vi "GetLeCroy_SynthFocus_25.vi"(1 "Digitizer Settings":T4={"Digitizer delay (us) "=0.0, "rf points per line"=2048, "lines per plane"=128, "Samp Rate (Hz)"=100000000.0, "Additional dig delay (us)"=0.0, "Voltage Scale"=0.4, "Pre-Looks"=0, "Offset delay (us)"=0.0, "bits A/D"=8, "Avg Num"=1, "DigTimeOut"=5.0, "Rel Dig Delay"=0.0, "Dig Ch"=0, "LeCroyCluster"={"LeCroy Channels"=[TRUE, FALSE, FALSE, FALSE], "LC read pt offset"=0.0, "Sweep Avg"=FALSE}, "Main Digitizer"=enum."NI Digitizer", "Dig Config"=enum."Single channel", "Digitizer ID Cluster"={"Acqiris/Alazar/SP ID"=[], "NI Instr Handles"=[], "LeCroy VISA"="", "GaGe Handle"={"Handle"=0, "Sample size"=0, "Resolution"=0, "Offset"=0, "Channels"=0, "Boards"=0}, "ATS Ref"="ATS9350", "Acqiris Address"=["PCI::INSTR0"], "ADQRef"=refnum, "adq_cu_ptr"=refnum}, "Trigger Settings"={"Trig Source"=1, "Trig Coupling"=0, "Trig Slope"=0, "Level (mV)"=1500.0}, "Bulk Acq"=FALSE, "Bulk Start Indexes"=[], "Data Ref RF"=refnum, "NI ID/Channel"=[], "Total Dig CH"=1, "Xtra Ann Trig delay (us)"=10.0, "Fix Z Delay?"=FALSE, "One Way Transmission?"=FALSE, "Data Ref Log"=refnum} {"Trigger Settings"."Trig Slope" items=["Positive", "Negative"]; "Trigger Settings"."Level (mV)" format="%.2f"; "Trigger Settings"."Trig Coupling" items=["DC 1 MOhm", "AC 1 MOhm", "DC 50 Ohm", "AC 50 Ohm"]; "Trigger Settings"."Trig Source" items=["Chan 1", "External"]; "Rel Dig Delay" format="%.2f"; "DigTimeOut" format="%.2f"; "Avg Num" min=1; "Offset delay (us)" format="%.2f"; "Additional dig delay (us)" format="%.2f"; "Digitizer delay (us)" format="%.2f"}, 5 "errorin":errorcluster, 6 "File Array":string[](array[string]), 7 "Ann Array Params":T1={"Synth Foc?"=FALSE, "Focal Zones"=41, "Switch T/R"=0, "Trans Geometry (mm)"={"Transducer"=0, "Geo Focus"=12.0, "a (radius)"=3.0, "# of rings"=5, "kerf space "=0.1, "Center Freq"=12.0}, "Sub Ap Excite?"=FALSE, "Full Array Scan?"=FALSE, "Xmt/Rcv"={"XMIT"=[TRUE, TRUE, TRUE, TRUE, TRUE], "RCV"=[TRUE, TRUE, TRUE, TRUE, TRUE]}, "PulseSpacing (us)"=0.0, "Xmit Ring"=0, "XMIT CHS"=0, "RCV CHS"=0, "GPU?"=FALSE, "Save TIFF?"=FALSE, "downfactor"=1, "RCV 1CH"=0} {"RCV 1CH" items=["All", "1", "2", "3", "4", "5"]; "Trans Geometry (mm)"."Transducer" items=["6D 12R 40 MHz"=0, "10D 31R 20 MHz"=1, "10D 23R 20 MHz"=2, "6D 23R 40 MHz"=3, "4.5D 10.7R 40 MHz"=4, "9D 23.5R 20 MHz"=5, "9D 25.8R 20MHz"=6, "Enter"=99]; "Switch T/R" min=1 max=5 step=1}, 8 "lines per plane":i32, 11 "Reverse?":bool) -> (12 "Gain Array":T8(array[cluster]), 13 "Raw VGain (scale)":dbl, 15 "VGain (dB)":dbl, 19 "error out":errorcluster)   [LabVIEW 2022 SP3]
uses:
  -DigitizerRoutines/DigitizerSettings.ctl
  -DigitizerRoutines/Digitizer.ctl
  -DigitizerRoutines/DigConfig.ctl
  -DigitizerRoutines/DigitizerID.ctl
  C:/Windows/System32/ADQAPI_dotNet_helper.dll
  Annular Array/-AnnularRoutines/AnnularArray.ctl
  Annular Array/-AnnularRoutines/TransGeometry.ctl
  Annular Array/-AnnularRoutines/ArrayGeometry.ctl
  Motion Controllers/-MotionRoutines/MotionGlobals.vi
  Annular Array/-SynthApperture/ProcImageHD_I16.vi
panel:
  out "read time":u32
  out "save time":u32
  out "Numeric":i32
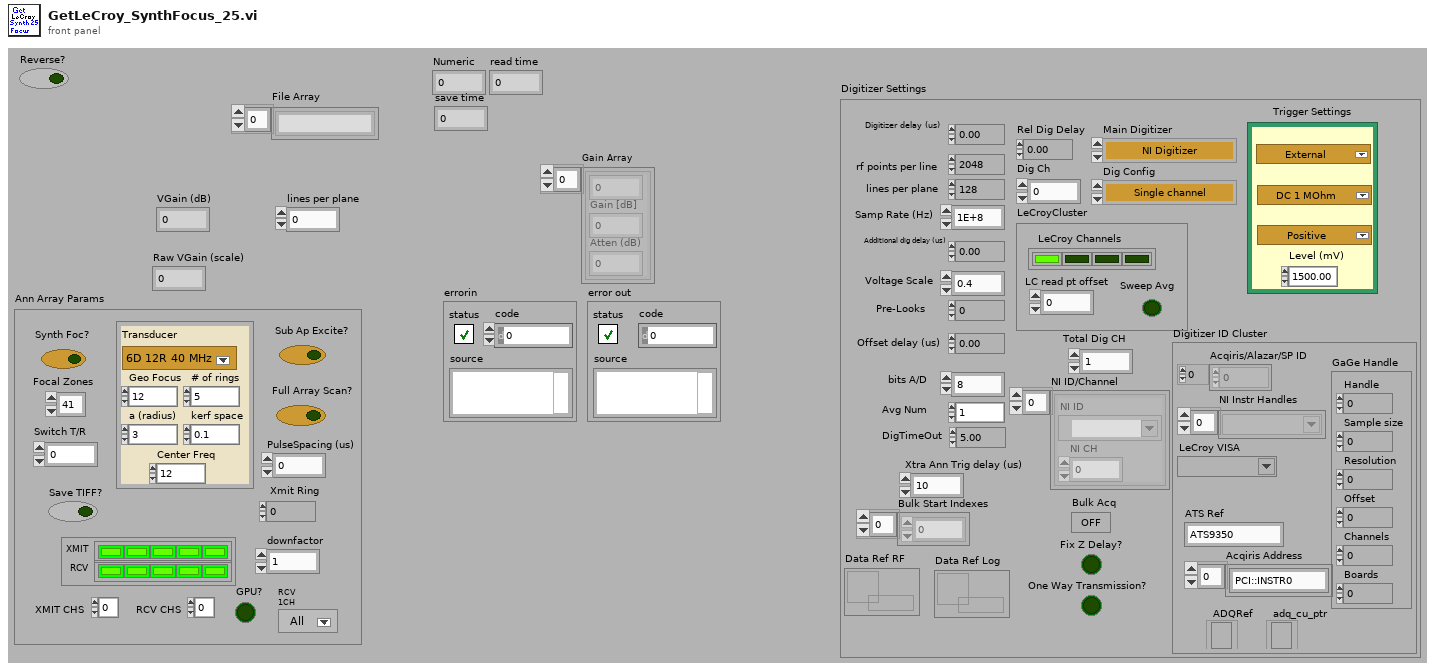
[diagram p1: front panel]
types:
  T1 = typedef "AnnularArray.ctl" = cluster{"Synth Foc?":bool, "Focal Zones":i16, "Switch T/R":i16, "Trans Geometry (mm)":T2, "Sub Ap Excite?":bool, "Full Array Scan?":bool, "Xmt/Rcv":cluster{"XMIT":bool[], "RCV":bool[]}, "PulseSpacing (us)":sgl, "Xmit Ring":i32, "XMIT CHS":u8, "RCV CHS":u8, "GPU?":bool, "Save TIFF?":bool, "downfactor":i32, "RCV 1CH":u16}
  T2 = typedef "TransGeometry.ctl" = cluster{"Transducer":T3, "Geo Focus":dbl, "a (radius)":dbl, "# of rings":i32, "kerf space ":dbl, "Center Freq":dbl}
  T3 = typedef "ArrayGeometry.ctl" = u16
  T4 = typedef "DigitizerSettings.ctl" = cluster{"Digitizer delay (us) ":dbl, "rf points per line":i32, "lines per plane":i32, "Samp Rate (Hz)":dbl, "Additional dig delay (us)":dbl, "Voltage Scale":dbl, "Pre-Looks":i32, "Offset delay (us)":dbl, "bits A/D":i8, "Avg Num":i32, "DigTimeOut":sgl, "Rel Dig Delay":sgl, "Dig Ch":i32, "LeCroyCluster":cluster{"LeCroy Channels":bool[], "LC read pt offset":dbl, "Sweep Avg":bool}, "Main Digitizer":T5, "Dig Config":T6, "Digitizer ID Cluster":T7, "Trigger Settings":cluster{"Trig Source":u16, "Trig Coupling":u16, "Trig Slope":u16, "Level (mV)":dbl}, "Bulk Acq":bool, "Bulk Start Indexes":i32[], "Data Ref RF":refnum<data-value>, "NI ID/Channel":cluster{"NI ID":refnum<k15>, "NI CH":i32}[], "Total Dig CH":i32, "Xtra Ann Trig delay (us)":dbl, "Fix Z Delay?":bool, "One Way Transmission?":bool, "Data Ref Log":refnum<data-value>}
  T5 = typedef "Digitizer.ctl" = enum16{"Acqiris Digitizer", "NI Digitizer", "LeCroy", "GaGe", "AlazarTech", "No Digitizer", "Teledyne"}
  T6 = typedef "DigConfig.ctl" = enum16{"Single channel", "2 Chans w/ 2 Acqiris", "2 Chans w/ 1 Acqiris", "5-CH Pulser New", "5-CH pulser w/ ann array", "5-pass style ann array", "Empty"}
  T7 = typedef "DigitizerID.ctl" = cluster{"Acqiris/Alazar/SP ID":u32[], "NI Instr Handles":refnum<k15>[], "LeCroy VISA":refnum<visa-resource-name>, "GaGe Handle":cluster{"Handle":u32, "Sample size":u32, "Resolution":i32, "Offset":i32, "Channels":u32, "Boards":u32}, "ATS Ref":string, "Acqiris Address":string[], "ADQRef":refnum<k24>, "adq_cu_ptr":refnum<k24>}
  T8 = cluster{sgl, "Gain [dB]  ":sgl, "Atten (dB)":sgl}[]
  T9 = cluster{"wfm":i16[][], "max queue size (-1, unlimited)":i32}
  T10 = cluster{"low cutoff":i32, "order":i32, "high cutoff":i32}
  T11 = cluster{sgl, "Gain [dB]  ":sgl, "Atten (dB)":sgl}
  T12 = cluster{"FIR Windowed Coefficients":dbl[], "Filter Prams":cluster{"low cutoff":i32, "order":i32, "high cutoff":i32}}
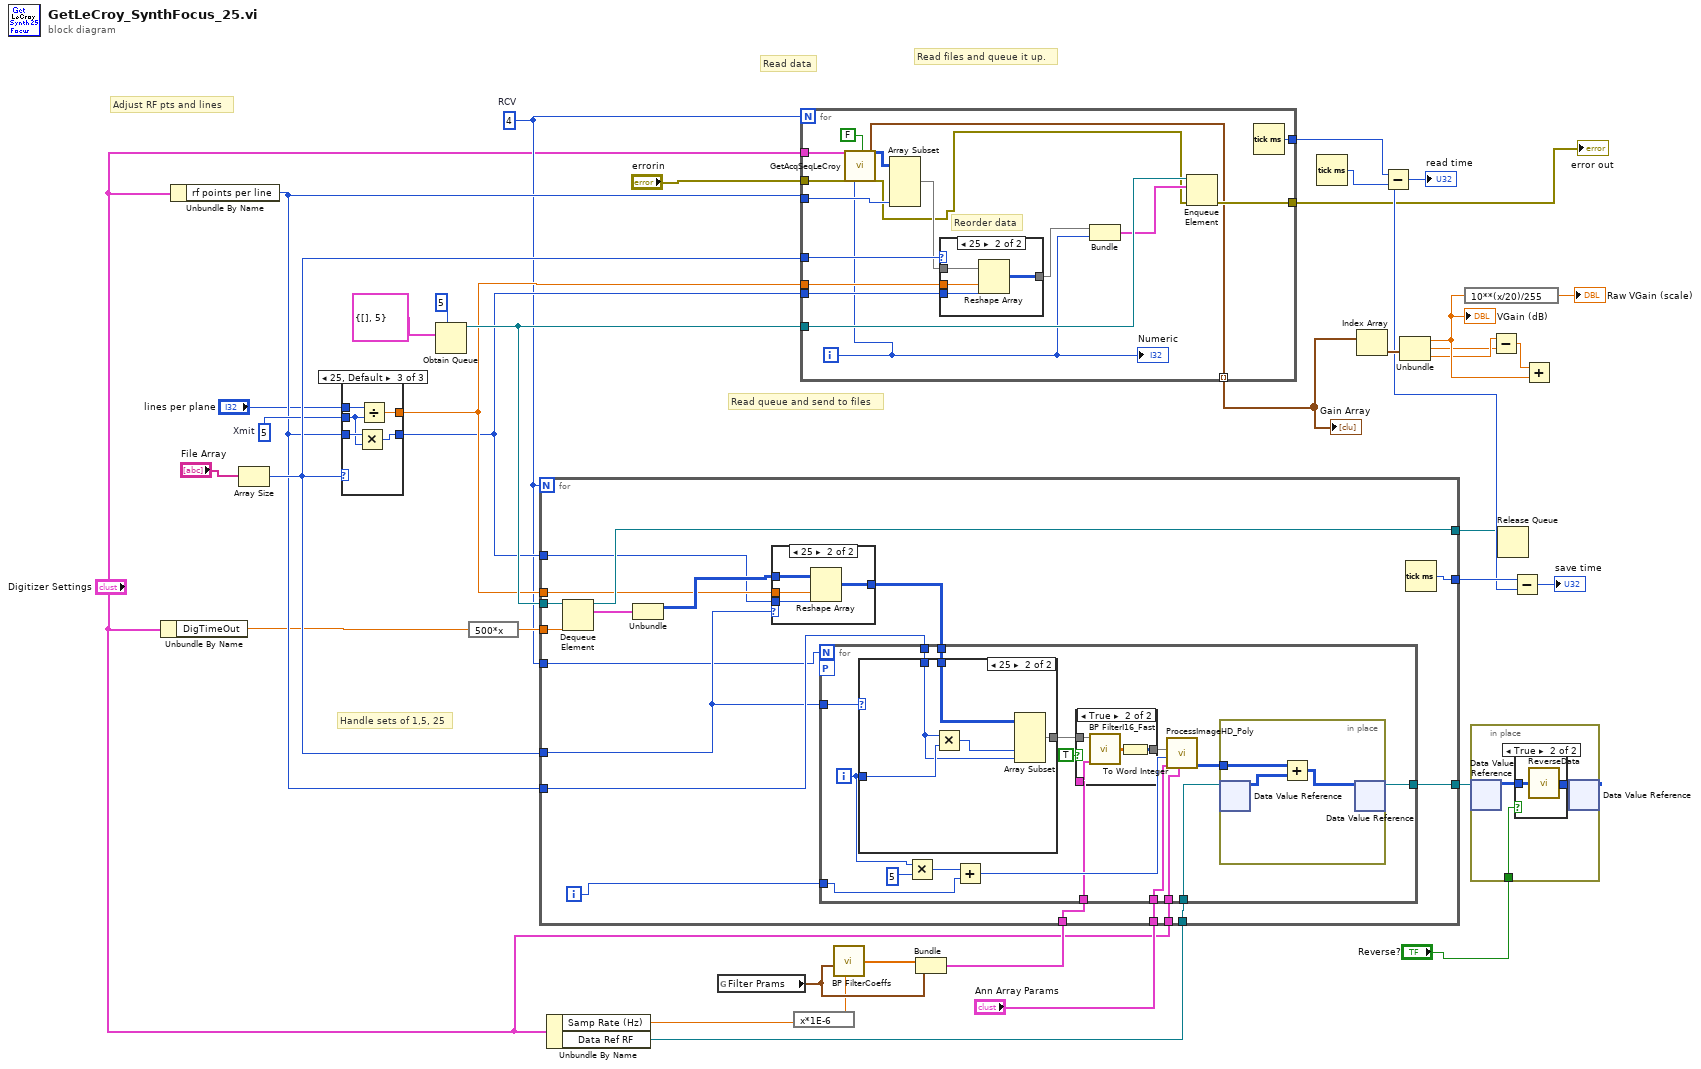
[diagram p0: block diagram]
diagram:
  w20 = 5  # Xmit
  w3 = 4  # RCV
  # "Read data"
  # "Adjust RF pts and lines"
  # "Handle sets of 1,5, 25"
  # "Read files and queue it up."
  # "Read queue and send to files"
  n1 = Unbundle By Name("Digitizer Settings") -> ("DigTimeOut"=w6:sgl)
  n2 = Unbundle By Name("Digitizer Settings") -> ("rf points per line"=w12:i32)
  n3 = Array Size(array="File Array") -> (size(s)=w21:i32)
  n4 = case shown="25, Default" w21 {
    tunnel: [w40 w42 w44] -> w18
    tunnel: w12 -> [w40 w42 w45]
    tunnel: [w39 w41 w46] -> w19
    tunnel: "lines per plane" -> [w39 w41 w47]
    tunnel: w20 -> [_ _ w43]
    frame 1 {
    }
    frame 5 {
    }
    frame 25, Default {
      n5 = Multiply(x=w45, y=w43) -> (x*y=w44:i32)
      n6 = Divide(x=w47, y=w43) -> (x/y=w46:dbl)
    }
  }
  n7 = Obtain Queue(max queue size (-1, unlimited)=5, element data type=T9 {"wfm"=[], "max queue size (-1, unlimited)"=5}) -> (queue out=w31:refnum<queue>)  [unwired: 3 in, 2 out]
  n8 = expression code="500*x"(w6) -> (w22:sgl)
  n9 = Unbundle By Name("Digitizer Settings") -> ("Samp Rate (Hz)"=w13:dbl, "Data Ref RF"=w11:refnum<data-value>)
  n10 = global read "MotionGlobals.vi" "Filter Prams"() -> (w17:T10)
  n11 = expression code="x*1E-6"(w13) -> (w16:dbl)
  n12 = for {
    N: w3 -> [_]
    tunnel: w31 -> [w64]
    tunnel: [w62] -> w29
    tunnel: [w61] -> w5
    tunnel: w21 -> [w60]
    tunnel: w19 -> [w59]
    tunnel: w18 -> [w58]
    tunnel: w12 -> [w56]
    tunnel: "errorin" -> [w54]
    tunnel: "Digitizer Settings" -> [w50]
    tunnel: [w48] -> w1 mode=indexing
    i -> [w52]
    # "Reorder data"
    n13 = call "GetAcqSeqLeCroy.vi"("Digitizer Settings"=w50, "errorin"=w54, "Source (0: Channel 1)"=w52, "save?"=FALSE) -> ("Voltage Scale"=w48:T11, "Data Array"=w53:i16[][], "error out"=w49:errorcluster)  [unwired: 17 in, 4 out]
    n14 = Array Subset(array=w53, length (col)=w56) -> (w55:i16[][])  [unwired: 3 in]
    n15 = case shown="25" w60 {
      tunnel: w58 -> [_ w69]
      tunnel: w55 -> [w65 w68]
      tunnel: [w65 w67] -> w57
      tunnel: w59 -> [_ w66]
      frame 0, Default {
      }
      frame 25 {
        n16 = Reshape Array(w68, w66, w69) -> (w67:i16[][])
      }
    }
    n17 = Bundle(w57, w52) -> (w63:cluster{i16[][], i32})  [unwired: 1 in]
    n18 = Enqueue Element(queue=w64, element=w63, error in (no error)=w49) -> (error out=w61:errorcluster)  [unwired: 1 in, 2 out]
    n19 = Tick Count (ms)() -> (millisecond timer value=w62:u32)
    "Numeric" <- w52
  }
  "error out" <- w5
  "Gain Array" <- w1
  n20 = call "BP FilterCoeffs.vi"("sample rate MHz"=w16, "Filter Prams"=w17) -> ("FIR Windowed Coefficients"=w15:dbl[])  [unwired: 4 in]
  n21 = Bundle("FIR Windowed Coefficients"=w15, "Filter Prams"=w17) -> (w14:T12)  [unwired: 1 in]
  n22 = for {
    N: w3 -> [_]
    tunnel: w12 -> [w78]
    tunnel: w31 -> [w87]
    tunnel: [w85] -> w24
    tunnel: [w84] -> w28
    tunnel: w21 -> [w77]
    tunnel: w22 -> [w83]
    tunnel: w19 -> [w81]
    tunnel: w18 -> [w80]
    tunnel: w14 -> [w76]
    tunnel: w11 -> [w75]
    tunnel: w3 -> [w73]
    tunnel: "Digitizer Settings" -> [w72]
    tunnel: "Ann Array Params" -> [w71]
    tunnel: [w70] -> w9
    i -> [w74]
    n23 = Dequeue Element(queue=w87, timeout in ms (-1)=w83) -> (queue out=w85:refnum<queue>, element=w86:T9)  [unwired: 1 in, 2 out]
    n24 = Unbundle(w86) -> ("wfm"=w82:i16[][])  [unwired: 1 out]
    n25 = case shown="25" w77 {
      tunnel: w80 -> [_ w123]
      tunnel: w82 -> [w119 w122]
      tunnel: [w119 w121] -> w79
      tunnel: w81 -> [_ w120]
      frame 0, Default {
      }
      frame 25 {
        n26 = Reshape Array(w122, w120, w123) -> (w121:i16[][])
      }
    }
    n27 = for {
      N: w73 -> [_]
      tunnel: w78 -> [w104]
      tunnel: w79 -> [w103]
      workers-P: _ -> [_]
      tunnel: w77 -> [w102]
      tunnel: w75 -> [w96]
      tunnel: w76 -> [w93]
      tunnel: w74 -> [w91]
      tunnel: w72 -> [w90]
      tunnel: w71 -> [w89]
      tunnel: [w88] -> w70
      i -> [w101]
      n28 = case shown="25" w102 {
        tunnel: [w113 w114] -> w95
        tunnel: w101 -> [_ w118]
        tunnel: w104 -> [_ w116]
        tunnel: w103 -> [w113 w115]
        frame 5, Default {
        }
        frame 25 {
          n29 = Multiply(x=w116, y=w118) -> (x*y=w117:i32)
          n30 = Array Subset(array=w115, index (col)=w117, length (col)=w116) -> (w114:i16[][])  [unwired: 2 in]
        }
      }
      n31 = Multiply(x=w101, y=5 ("max queue size (-1, unlimited)")) -> (x*y=w99:i32)
      n32 = Add(x=w99, y=w91) -> (x+y=w98:i32)
      n33 = case shown="True" TRUE {
        tunnel: w95 -> [w105 w108]
        tunnel: [w105 w107] -> w94
        tunnel: w93 -> [_ w106]
        frame False {
        }
        frame True {
          n34 = call "BP FilterI16_Fast.vi"("Filter"=w106, "Array in"=w108) -> ("Filtered X"=w109:dbl[][])  [unwired: 4 in]
          n35 = To Word Integer(number=w109) -> (16bit integer=w107:i16[][])
        }
      }
      n36 = call-poly "ProcessImageHD_Poly.vi"("Digitizer Settings"=w90, "Ann Array Params"=w89, "T/R Ring"=w98, "Scan Data In"=w94) -> ("Synth App Out"=w97:i16[][])  [unwired: 4 in, 1 out]
      n37 = in-place {
        in-place-border: w97 -> [w110]
        n38 = in-place-dvr #1(w96) -> (w112:i16[][])  [unwired: 1 out]
        n39 = Add(x=w110, y=w112) -> (x+y=w111:i16[][])
        n40 = in-place-dvr #1(w111) -> (w88:refnum<data-value>)  [unwired: 1 out]
      }
    }
    n41 = Tick Count (ms)() -> (millisecond timer value=w84:u32)
  }
  n42 = Tick Count (ms)() -> (millisecond timer value=w27:u32)
  n43 = Index Array(array=w1) -> (element=w38:T11)  [unwired: 1 in]
  n44 = Subtract(x=w29, y=w27) -> (x-y=→"read time":u32)
  n45 = Unbundle(w38) -> (w37:sgl, "Gain [dB]"=w35:sgl, "Atten (dB)"=w36:sgl)
  "VGain (dB)" <- w37
  n46 = expression code="10**(x/20)/255"(w37) -> (→"Raw VGain (scale)":sgl)
  n47 = in-place {
    in-place-border: "Reverse?" -> [w124]
    n48 = in-place-dvr #2(w9) -> (w126:i16[][])  [unwired: 1 out]
    n49 = case shown="True" w124 {
      tunnel: w126 -> [w127 w129]
      tunnel: [w127 w128] -> w125
      frame False {
      }
      frame True {
        n50 = call "ReverseData.vi"("Array in"=w129) -> ("Array out"=w128:i16[][])
      }
    }
    n51 = in-place-dvr #2(w125) -> ()  [unwired: 2 out]
  }
  n52 = Subtract(x=w36, y=w35) -> (x-y=w34:sgl)
  n53 = Release Queue(queue=w24) -> ()  [unwired: 2 in, 3 out]
  n54 = Subtract(x=w28, y=w27) -> (x-y=→"save time":u32)
  n55 = Add(x=w34, y=w37) -> ()  [unwired: 1 out]
